vi "Move Forward.vi"(11 "Are we using encoder?":bool) -> ()   [LabVIEW 2020]
uses:
  <vilib>/Rock Robotics/WPI/Utilities/WPI_GetSetVariantRefNum.vi
  Auto Variables.vi
  <vilib>/Rock Robotics/WPI/RobotDrive/WPI_RobotDriveArcadeDrive_Standard(NoSaturation).vi
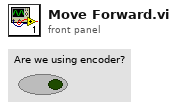
[diagram p1: front panel]
types:
  T1 = typedef "WPI_RobotDriveDevRef.ctl" = cluster{"DevStatus":errorcluster, "Motors[]":T2[], "Square Inputs":bool, "Max Output":dbl}
  T2 = typedef "WPI_MotorControlDeviceRef.ctl" = cluster{"DeviceStatus":errorcluster, "Type":T3, "PWM":cluster{"PWM Channel":T4, "DeadBand":T5}, "CAN":cluster{"Device Number":u8, "SetOutput VI Ref":variant, "GetOutput VI Ref":variant, "Enable VI Ref":variant, "Disable VI Ref":variant, "Data":variant}, "Invert":bool, "DIO PWM":cluster{"PWM \"Enable\" Channel":T4, "DIOChannel":T6, "PWM Rate":dbl}}
  T3 = typedef "WPI_MotorControlType.ctl" = enum16{"PWM", "CAN", "DIO PWM"}
  T4 = typedef "FPGA_DIOPWMChannel.ctl" = enum8{"PWM 0", "PWM 1", "PWM 2", "PWM 3", "PWM 4", "PWM 5", "PWM 6", "PWM 7", "PWM 8", "PWM 9", "PWM MXP 0", "PWM MXP 1", "PWM MXP 2", "PWM MXP 3", "PWM MXP 4", "PWM MXP 5", "PWM MXP 6", "PWM MXP 7", "PWM MXP 8", "PWM MXP 9", "Invalid"}
  T5 = typedef "WPI_PWMDeadband.ctl" = cluster{"Name":string, "maxPositivePwm":i32, "minPositivePwm":i32, "centerPwm":i32, "maxNegativePwm":i32, "minNegativePwm":i32, "angularRange":u16}
  T6 = typedef "FPGA_DIOChannel.ctl" = enum8{"DIO 0", "DIO 1", "DIO 2", "DIO 3", "DIO 4", "DIO 5", "DIO 6", "DIO 7", "DIO 8", "DIO 9", "DIO MXP 0", "DIO MXP 1", "DIO MXP 2", "DIO MXP 3", "DIO MXP 4", "DIO MXP 5", "DIO MXP 6", "DIO MXP 7", "DIO MXP 8", "DIO MXP 9", "DIO MXP 10", "DIO MXP 11", "DIO MXP 12", "DIO MXP 13", "DIO MXP 14", "DIO MXP 15", "SPI Port CS1", "SPI Port CS2", "SPI Port CS3", "SPI Port MISO", "SPI Port MOSI", "Invalid"}
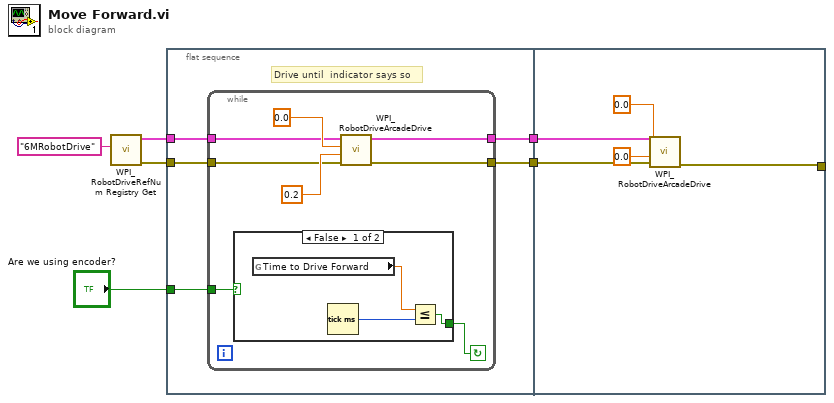
[diagram p0: block diagram]
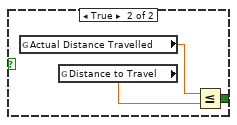
[diagram p2: hidden frame]
diagram:
  n1 = call <vilib>:"WPI_RobotDriveRefNum Registry Get.vi"("refnum name"="6MRobotDrive") -> ("error out"=w5:errorcluster, "RobotDriveDevRef"=w4:T1)  [unwired: 9 in]
  n2 = flat-sequence {
    tunnel: w5 -> [w11]
    tunnel: w4 -> [w10]
    tunnel: [w9] -> w3
    tunnel: [w8] -> w2
    tunnel: "Are we using encoder?" -> [w7]
    tunnel: w3 -> [w30]
    tunnel: w2 -> [w29]
    tunnel: [w26] -> _
    frame #0 {
      # "Drive until  indicator says so"
      n3 = while {
        tunnel: w11 -> [w17]
        tunnel: w10 -> [w16]
        tunnel: [w14] -> w9
        tunnel: [w13] -> w8
        tunnel: w7 -> [w12]
        stop <- w15 continue-if-true
        n4 = case shown="False" w12 {
          tunnel: [w22 w23] -> w15
          frame False {
            n5 = global read "Auto Variables.vi" "Time to Drive Forward"() -> (w21:dbl)
            n6 = Tick Count (ms)() -> (millisecond timer value=w20:u32)
            n7 = Less Or Equal?(x=w21, y=w20) -> (x <= y?=w22:bool)
          }
          frame True {
            n8 = global read "Auto Variables.vi" "Actual Distance Travelled"() -> (w25:dbl)
            n9 = global read "Auto Variables.vi" "Distance to Travel"() -> (w24:dbl)
            n10 = Less Or Equal?(x=w25, y=w24) -> (x <= y?=w23:bool)
          }
        }
        n11 = call-poly <vilib>:"WPI_RobotDriveArcadeDrive.vi"("error in (no error)"=w17, "Y axis value"=0.2, "X axis value"=0.0, "RobotDriveDevRef"=w16) -> ("error out"=w13:errorcluster, "RobotDriveDevRef"=w14:T1)  [unwired: 5 in, 1 out]
      }
    }
    frame #1 {
      n12 = call-poly <vilib>:"WPI_RobotDriveArcadeDrive.vi"("error in (no error)"=w29, "Y axis value"=0.0, "X axis value"=0.0, "RobotDriveDevRef"=w30) -> ("error out"=w26:errorcluster)  [unwired: 5 in, 2 out]
    }
  }
